vi "NewROI.vi"(11 "MagAnalysis_Online in":refnum<class "MagAnalysis_Online.lvclass">) -> (3 "MagAnalysis_Online out":refnum<class "MagAnalysis_Online.lvclass">)   [LabVIEW 2011, in "MagAnalysis_Online.lvclass"]
uses:
  MagAnalysis_Online.lvclass
  reshapeINfo_TypDef.ctl
  emptyArray_TYpDEf.ctl
  emptyArrayCamX_TypDef.ctl
  reshapeArrayCommand_TypDEf.ctl
  MagAnalysis_Online.lvclass/MagAnalysis_Online.ctl
  NI_AALBase.lvlib
panel:
  out "Array":dbl[](array[numeric])
  out "reshapeInfo":T1
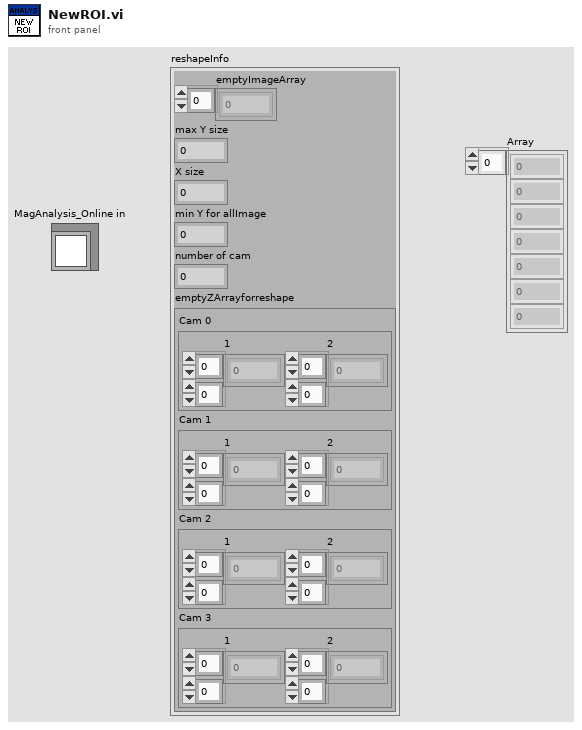
[diagram p1: front panel]
types:
  T1 = typedef "reshapeINfo_TypDef.ctl" = cluster{"emptyImageArray":dbl[], "max Y size":i32, "X size":i32, "min Y for allImage":dbl, "number of cam":i32, "emptyZArrayforreshape":T2}
  T2 = typedef "emptyArray_TYpDEf.ctl" = cluster{"Cam 0":T3, "Cam 1":T3, "Cam 2":T3, "Cam 3":T3}
  T3 = typedef "emptyArrayCamX_TypDef.ctl" = cluster{"1":dbl[][], "2":dbl[][]}
  T4 = cluster{"S 0":i32[][], "S 1":i32[][], "S 2":i32[][], "S 3":i32[][]}
  T5 = typedef "reshapeArrayCommand_TypDEf.ctl" = enum16{"init array", "addImage", "read", "init resolution"}
  T6 = typedef "CamSettings_Typdef.ctl" = cluster{"Cam 0":T7, "Cam 1":T7, "Cam 2":T7, "Cam 3":T7}
  T7 = typedef "CamSettingSUB_TypDEf.ctl" = cluster{"position":dbl, "Field of view":dbl, "start":dbl, "end":dbl, "center":dbl, "Lens":T8, "Forward":T9, "Spec_Calib_file 2":path, "map":path, "y size":i32}
  T8 = typedef "CamAndObj_TypDEf.ctl" = enum16{"FL1-f8x08", "FL1-f8x06", "FL1-f8", "ch300-f50", "FL2G-f8", "FL3M14-f8", "FL3M14-f8x08", "FL3M14-f8x08(2x2)"}
  T9 = typedef "OnOffTypeDef.ctl" = enum16{"off", "on"}
  T10 = typedef "Calib_Typdef.ctl" = cluster{"cam 0":T11, "cam 1":T11, "cam 2":T11, "cam 3":T11}
  T11 = typedef "calib_Sub_Typdef.ctl" = cluster{"incident ANGLE COMPENSATION":dbl[], "field of view /pixel":dbl, "dp/B [MeV/C/B]":dbl[], "charge compensation":dbl[], "Momentum [MeV/C]":dbl[], "B [T]":dbl, "energyDependence Input":dbl[], "pixel angle (y)":dbl[], "dp [MeV/C/] ":dbl[], "angle 2Dfor spectrumj":dbl[][], "dp [MeV/C] 2D":dbl[][], "charge compensation 2D":dbl[][], "Screen&Camera 2":T12, "ROI info":T13, "Y 2D full angle":dbl[][]}
  T12 = typedef "ScreenCam2_TypDEf.ctl" = cluster{"Screen Orientation":string, "Screen angle":string, "Lens":T8, "Calibration (mm/pix)":dbl}
  T13 = typedef "ROIInfo_TypDef.ctl" = cluster{"npix-X":i32, "npix-Y":i32, "Left [pix]":dbl, "Top [pix]":dbl}
  T14 = typedef "SrewMaster_TYpDef.ctl" = cluster{"Cam 0":T15, "Cam 1":T15, "Cam 2":T15, "Cam 3":T15}
  T15 = typedef "srew_TypDEf.ctl" = cluster{"S 0":T16, "S 1":T16, "S 2":T16, "S 3":T16, "S 4":T16, "S 5":T16}
  T16 = typedef "ScrewSub_Typdef.ctl" = cluster{"0":i32, "1":i32, "2":i32, "3":i32}
  T17 = typedef "screwstart.ctl" = cluster{"Cam 0":dbl, "Cam 1":dbl, "Cam 2":dbl, "Cam 3":dbl}
  T18 = cluster{"[0]":T11, "[1]":T11, "[2]":T11, "[3]":T11}
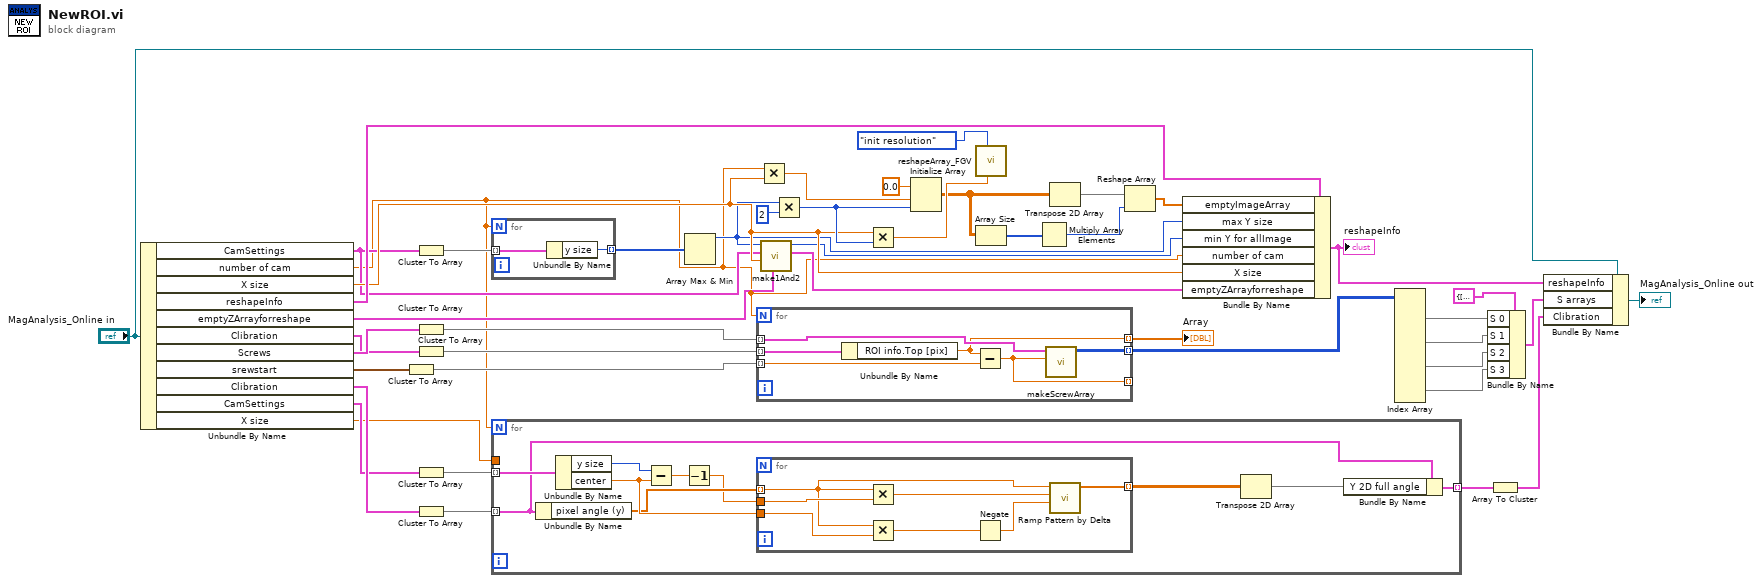
[diagram p0: block diagram]
diagram:
  n1 = Unbundle By Name("MagAnalysis_Online in") -> ("CamSettings"=w4:T6, "number of cam"=w1:dbl, "X size"=w31:dbl, "reshapeInfo"=w32:T1, "emptyZArrayforreshape"=w30:T2, "Clibration"=w9:T10, "Screws"=w18:T14, "srewstart"=w15:T17, "Clibration"=w12:T10, "CamSettings"=w8:T6, "X size"=w7:dbl)
  n2 = Cluster To Array(cluster=w15) -> (array=w14:dbl[])
  n3 = Cluster To Array(cluster=w4) -> (array=w3:T7[])
  n4 = Cluster To Array(cluster=w18) -> (array=w19:T15[])
  n5 = Cluster To Array(cluster=w9) -> (array=w17:T11[])
  n6 = Cluster To Array(cluster=w8) -> (array=w10:T7[])
  n7 = Cluster To Array(cluster=w12) -> (array=w11:T11[])
  n8 = for {
    N: w1 -> [_]
    tunnel: w3 -> [w47] mode=indexing
    tunnel: [w46] -> w2 mode=indexing
    n9 = Unbundle By Name(w47) -> ("y size"=w46:i32)
  }
  n10 = for {
    N: w1 -> [_]
    tunnel: w11 -> [w53] mode=indexing
    tunnel: w10 -> [w57] mode=indexing
    tunnel: w7 -> [_]
    tunnel: [w54] -> w6 mode=indexing
    n11 = Unbundle By Name(w53) -> ("pixel angle (y)"=w50:dbl[])
    n12 = Unbundle By Name(w57) -> ("y size"=w56:i32, "center"=w55:dbl)
    n13 = Subtract(x=w56, y=w55) -> (x-y=w49:dbl)
    n14 = Decrement(x=w49) -> (x-1=w48:dbl)
    n15 = for {
      tunnel: w50 -> [w61] mode=indexing
      tunnel: [w64] -> w51 mode=indexing
      tunnel: w48 -> [w63]
      tunnel: w55 -> [w62]
      n16 = Multiply(x=w61, y=w63) -> (x*y=w58:dbl)
      n17 = Multiply(x=w61, y=w62) -> (x*y=w60:dbl)
      n18 = Negate(x=w60) -> (-x=w59:dbl)
      n19 = call "Ramp Pattern by Delta.vi"("start"=w59, "end"=w58, "delta"=w61) -> ("Ramp Pattern"=w64:dbl[])  [unwired: 6 in, 2 out]
    }
    n20 = Transpose 2D Array(2D array=w51) -> (transposed array=w52:dbl[][])
    n21 = Bundle By Name(cluster=w53, "Y 2D full angle"=w52) -> (w54:T11)
  }
  n22 = Array Max & Min(array=w2) -> (max value=w26:i32)  [unwired: 3 out]
  n23 = for {
    N: w1 -> [_]
    tunnel: w17 -> [w70] mode=indexing
    tunnel: w19 -> [w69] mode=indexing
    tunnel: [w68] -> w25 mode=indexing
    tunnel: [w66] -> _ mode=indexing
    tunnel: w14 -> [w67] mode=indexing
    tunnel: [w65] -> w13 mode=indexing
    n24 = Unbundle By Name(w70) -> ("ROI info.Top [pix]"=w65:dbl)
    n25 = Subtract(x=w65, y=w67) -> (x-y=w66:dbl)
    n26 = call "makeScrewArray.vi"("start"=w66, "Cam 0"=w69) -> ("Array"=w68:i32[][])  [unwired: 9 in]
  }
  "Array" <- w13
  n27 = Multiply(x=w1, y=w31) -> (x*y=w39:dbl)
  n28 = call "make1And2.vi"("emptyZArrayforreshape in"=w30, "X size"=w31, "CamSettings"=w4, "MaxY"=w26) -> ("emptyZArrayforreshape out"=w29:T2, "min Y"=w27:i32)  [unwired: 6 in]
  n29 = Multiply(x=w26, y=2) -> (x*y=w42:i32)
  n30 = Multiply(x=w31, y=w42) -> (x*y=w43:dbl)
  n31 = Initialize Array(0.0, w39, w42) -> (w36:dbl[][])
  n32 = call "reshapeArray_FGV.vi"("single image size"=w43, "command"=reshapeArrayCommand_TypDEf."init resolution") -> ()  [unwired: 8 in, 2 out]
  n33 = Array Size(array=w36) -> (size(s)=w37:i32[])
  n34 = Multiply Array Elements(1:w37) -> (0:w38:i32)
  n35 = Transpose 2D Array(2D array=w36) -> (transposed array=w35:dbl[][])
  n36 = Reshape Array(w35, w38) -> (w33:dbl[])
  n37 = Bundle By Name(cluster=w32, "emptyImageArray"=w33, "max Y size"=w26, "min Y for allImage"=w27, "number of cam"=w1, "X size"=w31, "emptyZArrayforreshape"=w29) -> (w28:T1)
  "reshapeInfo" <- w28
  n38 = Index Array(array=w25) -> (element #1=w23:i32[][], element #2=w22:i32[][], element #3=w21:i32[][], element #4=w20:i32[][])  [unwired: 12 in]
  n39 = Bundle By Name(cluster=T4 {"S 0"=[], "S 1"=[], "S 2"=[], "S 3"=[]} ("S arrays"), "S 0"=w23, "S 1"=w22, "S 2"=w21, "S 3"=w20) -> (w16:T4)
  n40 = Array To Cluster(array=w6) -> (cluster=w5:T18)
  n41 = Bundle By Name(cluster="MagAnalysis_Online in", "reshapeInfo"=w28, "S arrays"=w16, "Clibration"=w5) -> (→"MagAnalysis_Online out":refnum<class "MagAnalysis_Online.lvclass">)
